vi "Cycle Count XML Default Text.vi"() -> (3 "Cycle Counter XML String":string)   [LabVIEW 2015, in "Tool Module.lvlib"]
doc: "<b>Note:</b> This VI was modified by the <b>Validate DQMH Module</b> tool to turn off automatic error handling."
uses:
  Tool Module.lvlib
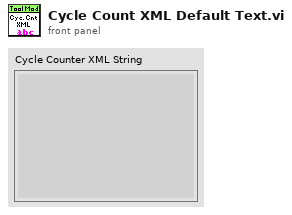
[diagram p1: front panel]
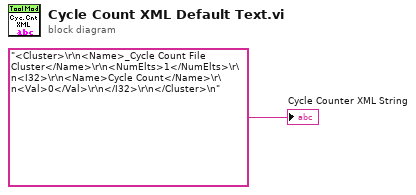
[diagram p0: block diagram]
diagram:
  "Cycle Counter XML String" <- "<Cluster>\r\n<Name>_Cycle Count File Cluster</Name>\r\n<NumElts>1</NumElts>\r\n<I32>\r\n<Name>Cycle Count</Name>\r\n<Val>0</Val>\r\n</I32>\r\n</Cluster>\n"
